vi "OutRefArray.vi"() -> ()   [LabVIEW 2015]
uses:
  <vilib>/Utility/miscctls.llb/LVPositionTypeDef.ctl
panel:
  out "RefArray":refnum<vi>[](array[refnum])
  out "RefNameArray":string[](array[string])
  in  "Boolean 7":bool=TRUE
  in  "Boolean 6":bool=TRUE
  in  "Boolean 5":bool=TRUE
  in  "Boolean 4":bool=TRUE
  in  "Boolean 3":bool=TRUE
  in  "Boolean 2":bool=TRUE
  out "RefClusterArray":T2(array[cluster])
  in  "Boolean":bool
  out "GObjArray":T3(array[cluster])
  in  "Numeric":dbl
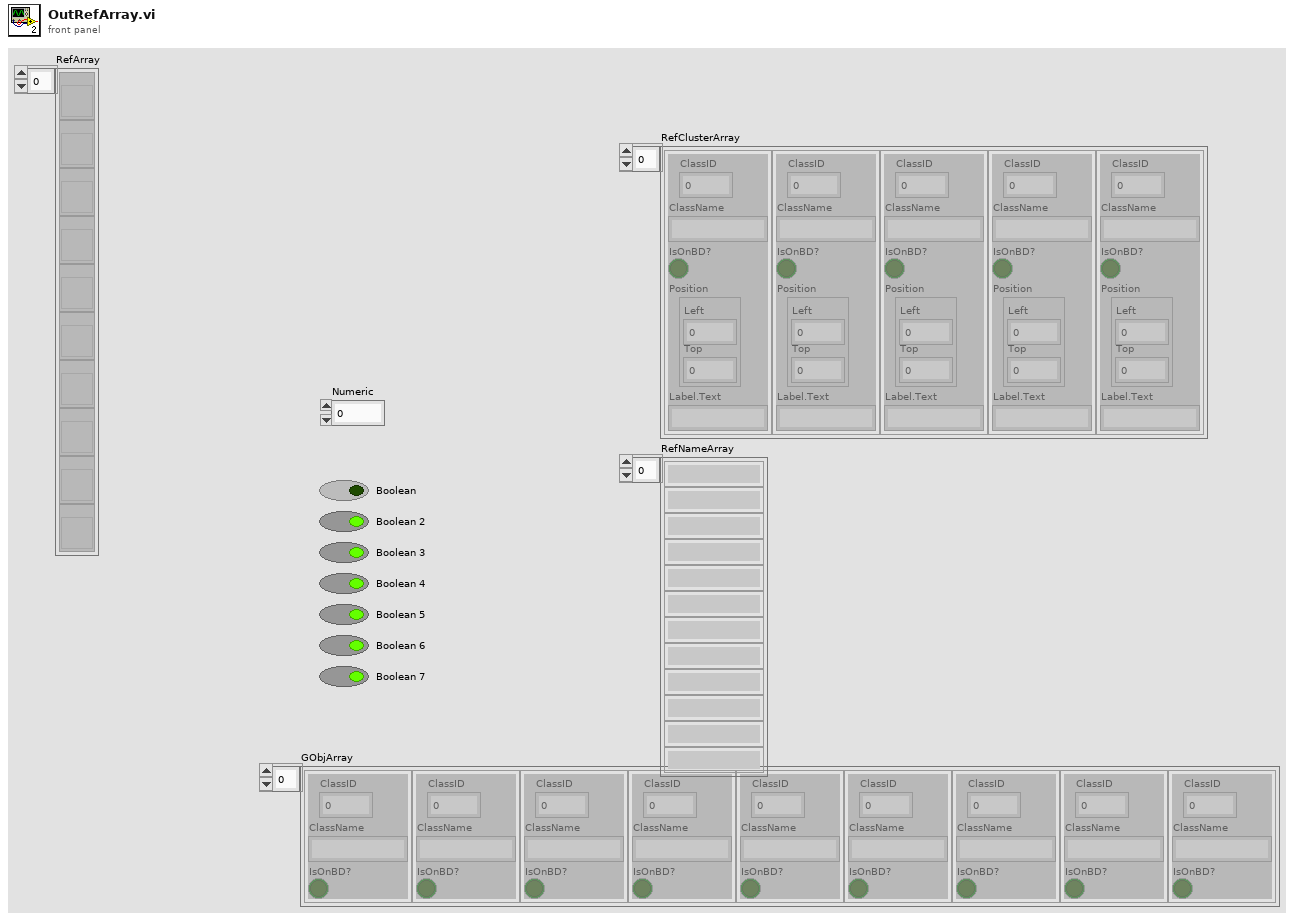
[diagram p1: front panel]
types:
  T1 = typedef "LVPositionTypeDef.ctl" = cluster{"Left":i32, "Top":i32}
  T2 = cluster{"ClassID":u32, "ClassName":string, "IsOnBD?":bool, "Position":T1, "Label.Text":string}[]
  T3 = cluster{"ClassID":u32, "ClassName":string, "IsOnBD?":bool}[]
  T4 = cluster{"ClassID":u32, "ClassName":string, "IsOnBD?":bool}
  T5 = cluster{"ClassID":u32, "ClassName":string, "IsOnBD?":bool, "Position":T1, "Label.Text":string}
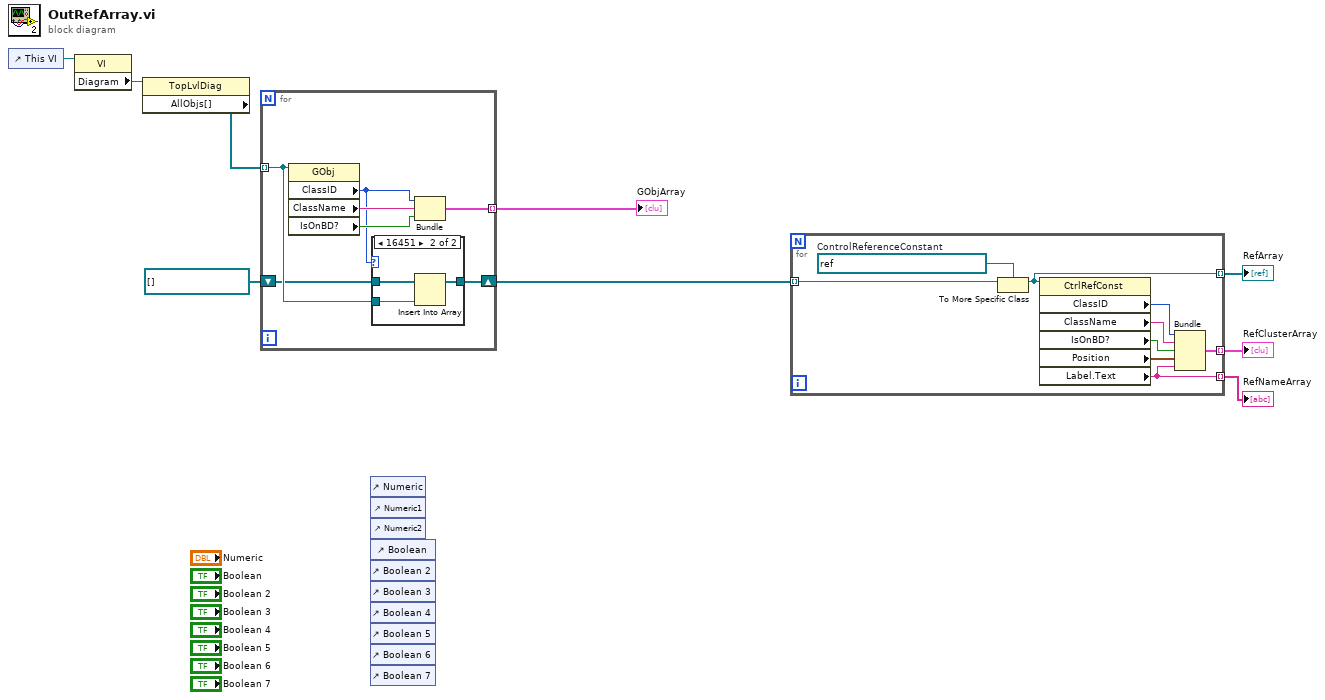
[diagram p0: block diagram]
diagram:
  n1 = control-ref of="This VI"() -> (w9:refnum<vi>)
  n2 = property class="VI"(reference=w9) -> ("Diagram"=w8:refnum<vi>)  [unwired: 1 in, 2 out]
  n3 = property class="TopLvlDiag"(reference=w8) -> ("AllObjs[]"=w7:refnum<vi>[])  [unwired: 1 in, 2 out]
  n4 = for {
    tunnel: w7 -> [w13] mode=indexing
    tunnel: [w14] -> w3 mode=indexing
    shift-right: [w12] -> w5
    shift-left: refnum<vi>[] [] -> [w11]
    n5 = property class="GObj"(reference=w13) -> ("ClassID"=w10:u32, "ClassName"=w16:string, "IsOnBD?"=w15:bool)  [unwired: 1 in, 2 out]
    n6 = case shown="16451" w10 {
      tunnel: w13 -> [_ w20]
      tunnel: [w17 w19] -> w12
      tunnel: w11 -> [w17 w18]
      frame 0, Default {
      }
      frame 16451 {
        n7 = Insert Into Array(array=w18, new element=w20) -> (w19:refnum<vi>[])  [unwired: 1 in]
      }
    }
    n8 = Bundle("ClassID"=w10, "ClassName"=w16, "IsOnBD?"=w15) -> (w14:T4)  [unwired: 1 in]
  }
  "GObjArray" <- w3
  n9 = control-ref of="Numeric"() -> ()  [unwired: 1 out]
  n10 = control-ref of="Numeric1"() -> ()  [unwired: 1 out]
  n11 = control-ref of="Numeric2"() -> ()  [unwired: 1 out]
  n12 = control-ref of="Boolean"() -> ()  [unwired: 1 out]
  n13 = control-ref of="Boolean 2"() -> ()  [unwired: 1 out]
  n14 = control-ref of="Boolean 3"() -> ()  [unwired: 1 out]
  n15 = control-ref of="Boolean 4"() -> ()  [unwired: 1 out]
  n16 = control-ref of="Boolean 5"() -> ()  [unwired: 1 out]
  n17 = control-ref of="Boolean 6"() -> ()  [unwired: 1 out]
  n18 = control-ref of="Boolean 7"() -> ()  [unwired: 1 out]
  n19 = for {
    tunnel: w5 -> [w24] mode=indexing
    tunnel: [w27] -> w4 mode=indexing
    tunnel: [w22] -> w2 mode=indexing
    tunnel: [w21] -> w1 mode=indexing
    w23 = refnum<vi> refnum  # ControlReferenceConstant
    n20 = To More Specific Class(target class=w23, reference=w24) -> (specific class reference=w21:refnum<vi>)  [unwired: 1 in, 1 out]
    n21 = property class="CtrlRefConst"(reference=w21) -> ("ClassID"=w26:u32, "ClassName"=w29:string, "IsOnBD?"=w28:bool, "Position"=w25:T1, "Label.Text"=w22:string)  [unwired: 1 in, 2 out]
    n22 = Bundle("ClassID"=w26, "ClassName"=w29, "IsOnBD?"=w28, "Position"=w25, "Label.Text"=w22) -> (w27:T5)  [unwired: 1 in]
  }
  "RefClusterArray" <- w4
  "RefNameArray" <- w2
  "RefArray" <- w1
